vi "Simple_Lag_Filter.vi"(10 "Input":dbl, 11 "Lag":dbl) -> (3 "Lagged Ouptut":dbl)   [LabVIEW 2019]
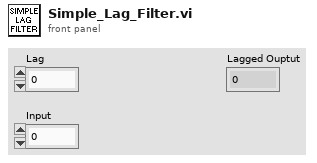
[diagram p1: front panel]
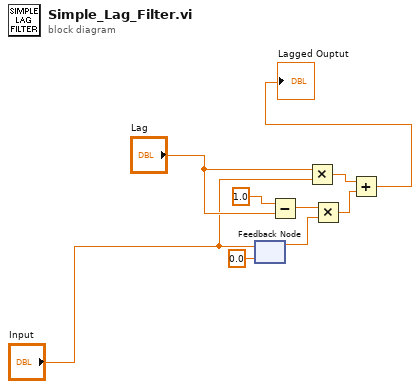
[diagram p0: block diagram]
diagram:
  n1 = feedback #1(0.0 ("Normalized Left Wheel Demand")) -> (w5:dbl)
  n2 = feedback-in #1("Input") -> ()
  n3 = Subtract(x=1.0, y="Lag") -> (x-y=w4:dbl)
  n4 = Multiply(x="Lag", y="Input") -> (x*y=w7:dbl)
  n5 = Multiply(x=w4, y=w5) -> (x*y=w8:dbl)
  n6 = Add(x=w7, y=w8) -> (x+y=→"Lagged Ouptut":dbl)
